vi "globalVariables.vi"() -> ()   [LabVIEW 2012]
uses:
  TimeValue.ctl
  SensorSettingCtl.ctl
panel:
  in  "test global var":u32
  in  "stop measurement":bool
  out "Saved Configuration":T1[](array[typedef])
  in  "AllValues":T2[][](array[typedef])
  in  "NewestValues":T2[](array[typedef])=[{"Time of measurement"=timestamp(0 s since 1904-01-01), "Current value"=0.0}, {"Time of measurement"=timestamp(0 s since 1904-01-01), "Current value"=0.0}, {"Time of measurement"=timestamp(0 s since 1904-01-01), "Current value"=0.0}, {"Time of measurement"=timestamp(0 s since 1904-01-01), "Current value"=0.0}, {"Time of measurement"=timestamp(0 s since 1904-01-01), "Current value"=0.0}]
  in  "MaxNrOfChannels":i32=5
  out "Errors":errorcluster[](array[cluster])
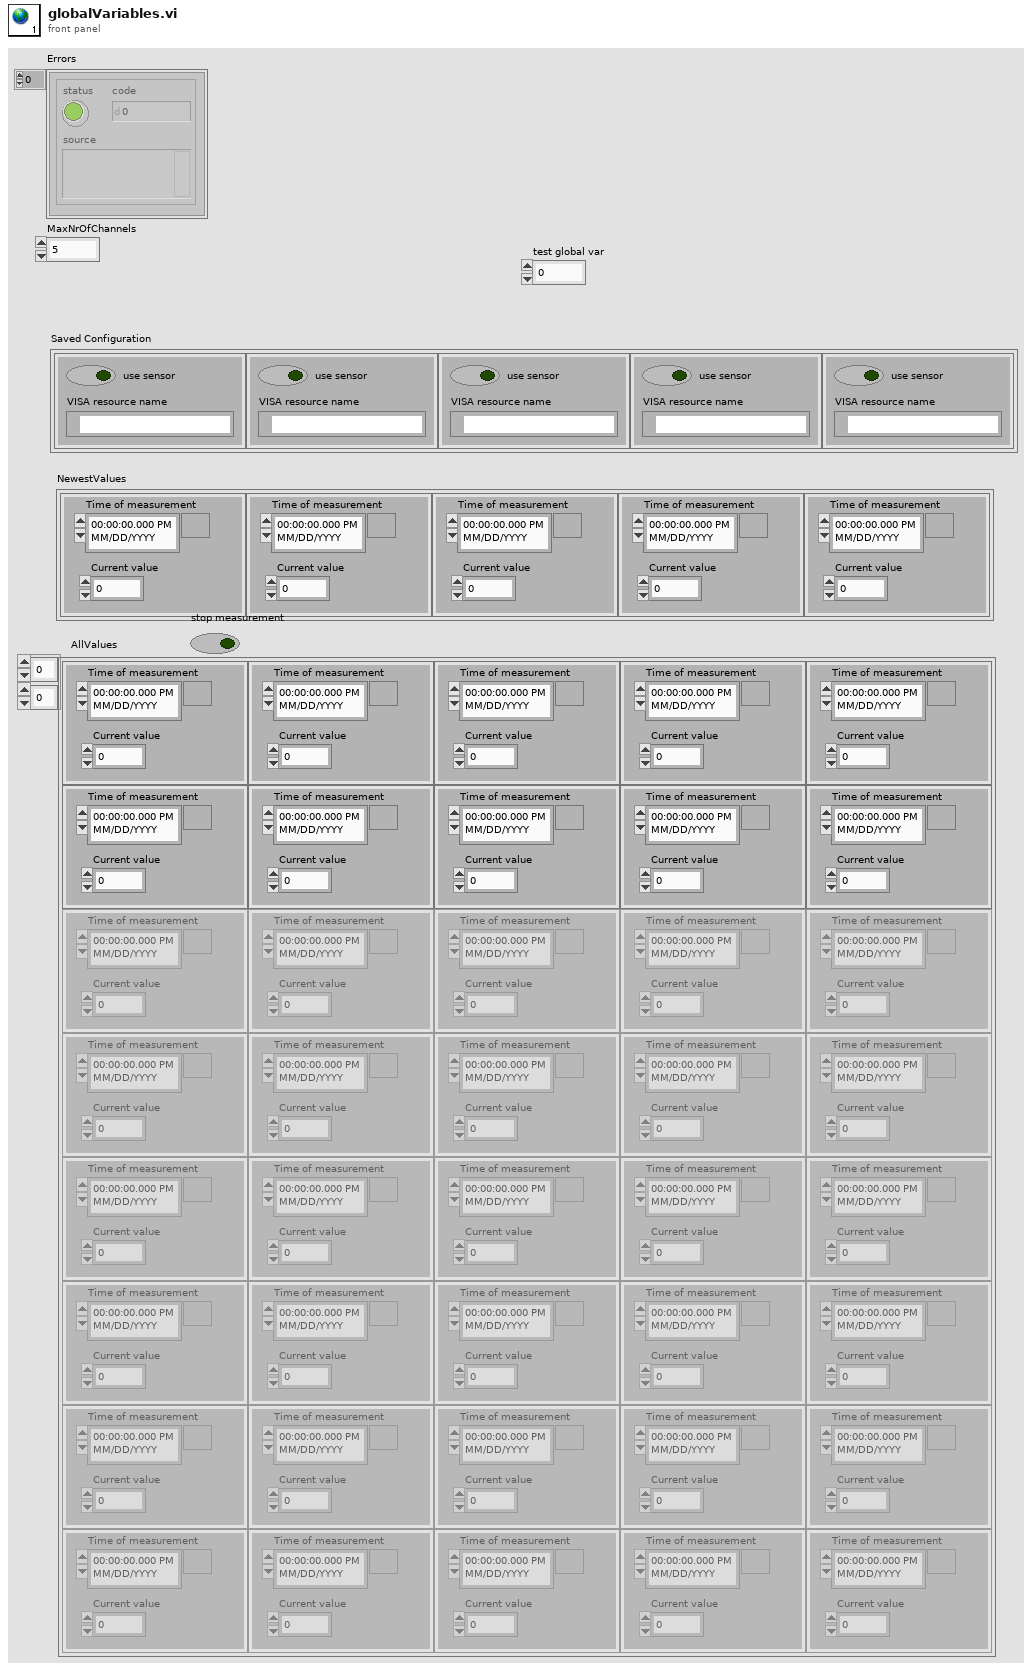
[diagram p1: front panel]
types:
  T1 = typedef "SensorSettingCtl.ctl" = cluster{"VISA resource name":refnum<visa-resource-name>, "use sensor":bool}
  T2 = typedef "TimeValue.ctl" = cluster{"Time of measurement":timestamp, "Current value":dbl}
diagram:
